vi "SwerveDriveLogic.vi"(9 "Speeds":dbl[](array[numeric]), 10 "AngleSetpoints":dbl[](array[numeric]), 11 "AngleEncoders":dbl[](array[numeric])) -> (2 "AngleMotorsReversed":bool[](array[boolean]), 3 "AngleMotorOutputs":dbl[](array[numeric]))   [LabVIEW 2018]
uses:
  <vilib>/Rock Robotics/Network Tables/NT Write Numeric Array.vi
  <vilib>/addons/control/pid/pid.llb/PID (DBL).vi
  <vilib>/Rock Robotics/Network Tables/NT Write Boolean Array.vi
  <vilib>/addons/control/pid/NI_PID_pid.lvlib
panel:
  out "Back right module":dbl(knob)
  out "Back left module":dbl(knob)
  out "Front left module":dbl(knob)
  out "Front right module":dbl(knob)
  in  "PID gains":T1={"proportional gain (Kc)"=0.05, "integral time (Ti, min)"=0.0, "derivative time (Td, min)"=0.0} {"derivative time (Td, min)" format="%.15f"; "integral time (Ti, min)" format="%.3f"; "proportional gain (Kc)" format="%.3f"}
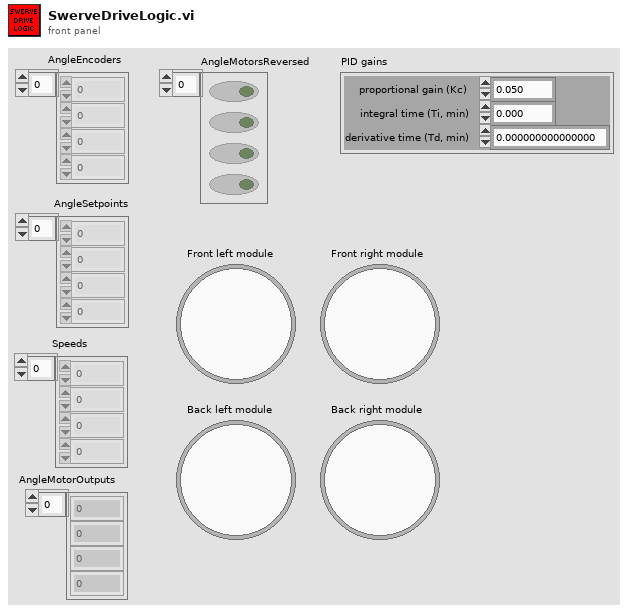
[diagram p1: front panel]
types:
  T1 = cluster{"proportional gain (Kc)":dbl, "integral time (Ti, min)":dbl, "derivative time (Td, min)":dbl}
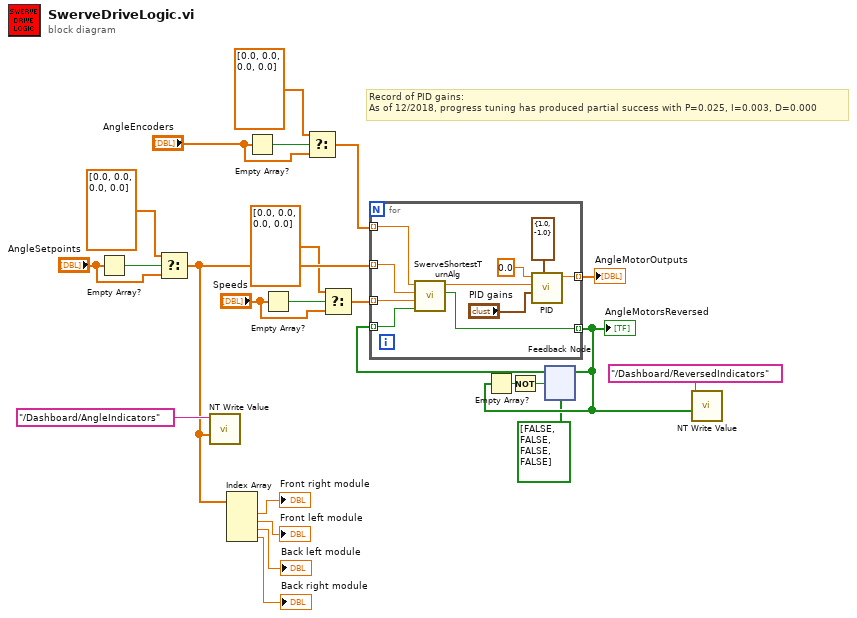
[diagram p0: block diagram]
diagram:
  # "Record of PID gains:\nAs of 12/2018, progress tuning has produced partial success with P=0.025, I=0.003, D=0.000"
  n1 = Empty Array?(array="AngleSetpoints") -> (empty?=w9:bool)
  n2 = Select(t=dbl[] [0.0, 0.0, 0.0, 0.0] ("AngleSetpoints"), s=w9, f="AngleSetpoints") -> (s? t:f=w7:dbl[])
  n3 = call-poly <vilib>:"NT Write Value.vi"("Numeric Array"=w7, "Name"="/Dashboard/AngleIndicators") -> ()  [unwired: 9 in, 1 out]
  n4 = Index Array(array=w7) -> (element #1=→"Front right module":dbl, element #2=→"Front left module":dbl, element #3=→"Back left module":dbl, element #4=→"Back right module":dbl)  [unwired: 4 in]
  n5 = Empty Array?(array="AngleEncoders") -> (empty?=w13:bool)
  n6 = Empty Array?(array="Speeds") -> (empty?=w5:bool)
  n7 = Select(t=dbl[] [0.0, 0.0, 0.0, 0.0] ("AngleSetpoints"), s=w13, f="AngleEncoders") -> (s? t:f=w10:dbl[])
  n8 = Select(t=dbl[] [0.0, 0.0, 0.0, 0.0] ("AngleSetpoints"), s=w5, f="Speeds") -> (s? t:f=w3:dbl[])
  n9 = feedback #1(bool[] [FALSE, FALSE, FALSE, FALSE]) -> (w15:bool[])
  n10 = for {
    tunnel: w15 -> [w27] mode=indexing
    tunnel: w7 -> [w30] mode=indexing
    tunnel: [w33] -> w24 mode=indexing
    tunnel: [w32] -> w16 mode=indexing
    tunnel: w10 -> [w26] mode=indexing
    tunnel: w3 -> [w25] mode=indexing
    n11 = call "SwerveShortestTurnAlg.vi"("SwerveMotorsFlipped?"=w27, "SwerveSpeed"=w25, "AngleSetpoint"=w30, "AngleEncoder"=w26) -> ("FlipSwerveMotors"=w32:bool, "PIDInput"=w29:dbl)  [unwired: 6 in]
    n12 = call-poly <vilib>:"PID.vi"("output range"=cluster{"output high":dbl, "output low":dbl} {"output high"=1.0, "output low"=-1.0}, "PID gains"="PID gains", "process variable"=w29, "setpoint"=0.0) -> ("output"=w33:dbl)  [unwired: 6 in, 1 out]
  }
  "AngleMotorOutputs" <- w24
  "AngleMotorsReversed" <- w16
  n13 = Empty Array?(array=w16) -> (empty?=w17:bool)
  n14 = Not(x=w17) -> (.not. x?=w1:bool)
  n15 = feedback-in #1(w16, w1) -> ()
  n16 = call-poly <vilib>:"NT Write Value.vi"("Boolean Array"=w16, "Name"="/Dashboard/ReversedIndicators") -> ()  [unwired: 9 in, 1 out]
